vi "inv_kin_test_pose.vi"() -> ()   [LabVIEW 2014]
uses:
  <vilib>/Analysis/Matrix/Datatypes/RealMatrix.ctl
  <vilib>/Analysis/Matrix/NI_Matrix.lvlib
panel:
  out "Failure":bool
  out "Pose vector out":dbl[](array[numeric]) format="%#.3f"
  out "Result pose":T1 format="%#_3p"
  out "RMS mismatch (mm/degree)":dbl
  out "number of function evaluations":i32
  out "Error":string
  out "f(minimum)":dbl
  out "Mismatch":dbl[](array[numeric]) format="%#_3g"
  out "Axis positions out":dbl[](array[numeric]) format="%#.3f"
  out "Pose":T1 format="%#_3p"
  in  "Pose XYZ Rx Ry Rz":dbl[](array[numeric])=[0.0, 0.0, 0.0, 0.0, 0.0, 0.0]
  # "RMS pose error (~microns)"
  # "Test inverse kinematics w.r.t. forward kinematics by starting with axis positions, converting to pose, then back again.  If there is gimbal lock, then there may be considerable mismatch in axis positions even though the pose is correct."
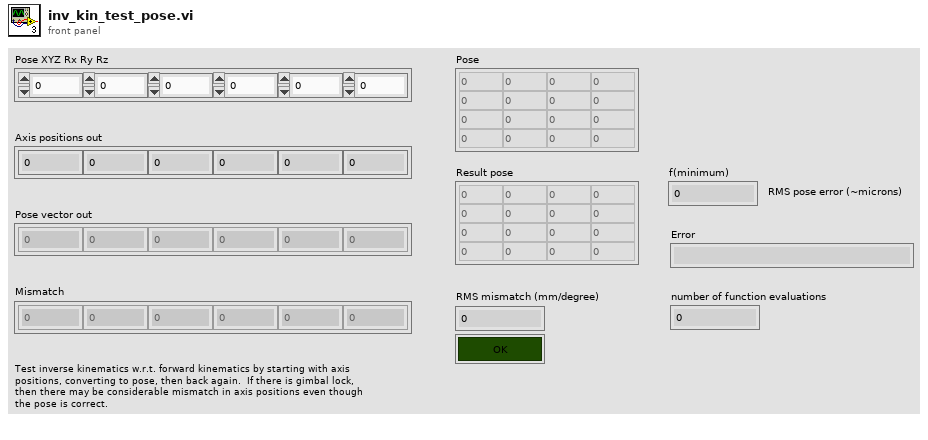
[diagram p1: front panel]
types:
  T1 = typedef "NI_Matrix.lvlib/RealMatrix.ctl" = dbl[][]
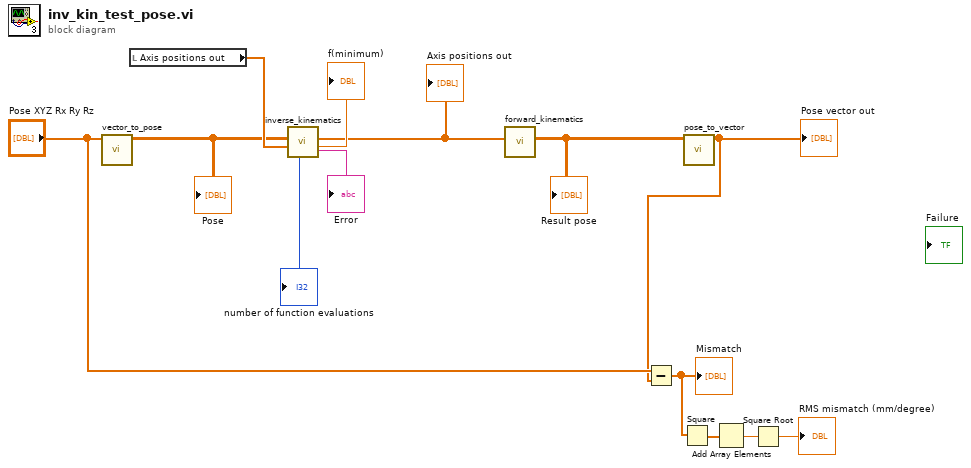
[diagram p0: block diagram]
diagram:
  n1 = call "vector_to_pose.vi"("Pose vector"="Pose XYZ Rx Ry Rz") -> ("Pose"=w5:T1)  [unwired: 10 in]
  "Pose" <- w5
  n2 = local read "Axis positions out"() -> (w6:dbl[])
  n3 = call "inverse_kinematics.vi"("Initial axis positions"=w6, "Pose"=w5) -> ("f(minimum)"=→"f(minimum)":dbl, "Axis positions"=w4:dbl[], "Error"=→"Error":string, "number of function evaluations"=→"number of function evaluations":i32)  [unwired: 5 in, 1 out]
  "Axis positions out" <- w4
  n4 = call "forward_kinematics.vi"("Axis positions"=w4) -> ("Pose"=w3:T1)  [unwired: 10 in]
  "Result pose" <- w3
  n5 = call "pose_to_vector.vi"("Pose"=w3) -> ("Pose vector"=w1:dbl[])  [unwired: 10 in]
  "Pose vector out" <- w1
  n6 = Subtract(x="Pose XYZ Rx Ry Rz", y=w1) -> (x-y=w8:dbl[])
  "Mismatch" <- w8
  n7 = Square(x=w8) -> (x^2=w9:dbl[])
  n8 = Add Array Elements(numeric array=w9) -> (sum=w10:dbl)
  n9 = Square Root(x=w10) -> (sqrt(x)=→"RMS mismatch (mm/degree)":dbl)
